vi "Set Results.vi"(8 "error in (no error)":errorcluster, 10 "Results":T1, 11 "niDTS GNSS Dut in":refnum<class "niDTS GNSS Dut.lvclass">) -> (0 "error out":errorcluster, 3 "niDTS GNSS Dut out":refnum<class "niDTS GNSS Dut.lvclass">)   [LabVIEW 2015, in "niDTS GNSS.lvlib" / "niDTS GNSS Dut.lvclass"]
uses:
  niDTS GNSS Dut.lvclass
  Tests/RF Test/Includes/niDTS GNSS RF Test INC Results.ctl
  niDTS GNSS Dut.lvclass/niDTS GNSS Dut.ctl
  niDTS GNSS.lvlib
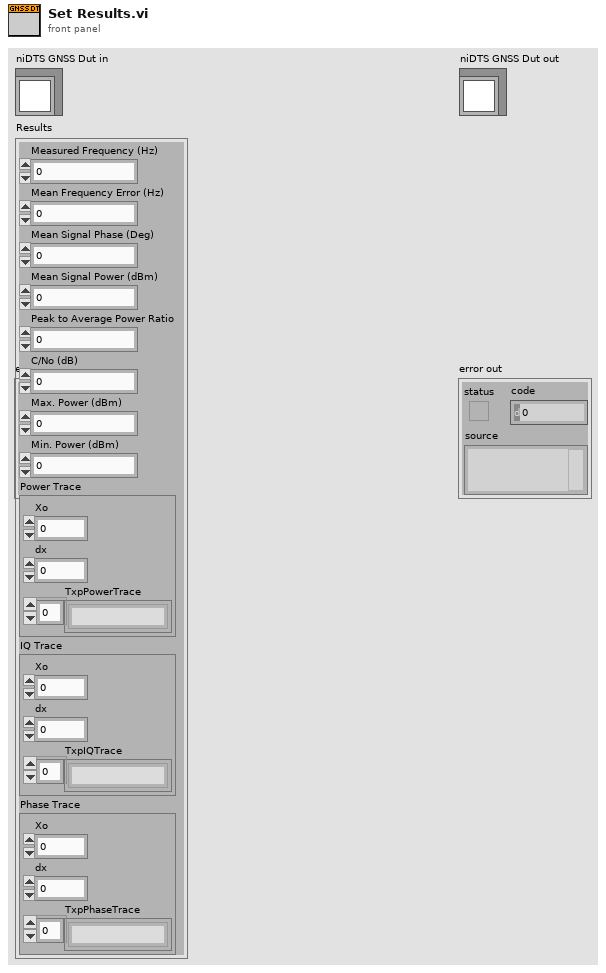
[diagram p1: front panel]
types:
  T1 = typedef "niDTS GNSS.lvlib/niDTS GNSS RF Test INC Results.ctl" = cluster{"Measured Frequency (Hz)":dbl, "Mean Frequency Error (Hz)":dbl, "Mean Signal Phase (Deg)":dbl, "Mean Signal Power (dBm)":dbl, "Peak to Average Power Ratio":dbl, "C/No (dB)":dbl, "Max. Power (dBm)":dbl, "Min. Power (dBm)":dbl, "Power Trace":cluster{"Xo":dbl, "dx":dbl, "TxpPowerTrace":string[]}, "IQ Trace":cluster{"Xo":dbl, "dx":dbl, "TxpIQTrace":string[]}, "Phase Trace":cluster{"Xo":dbl, "dx":dbl, "TxpPhaseTrace":string[]}}
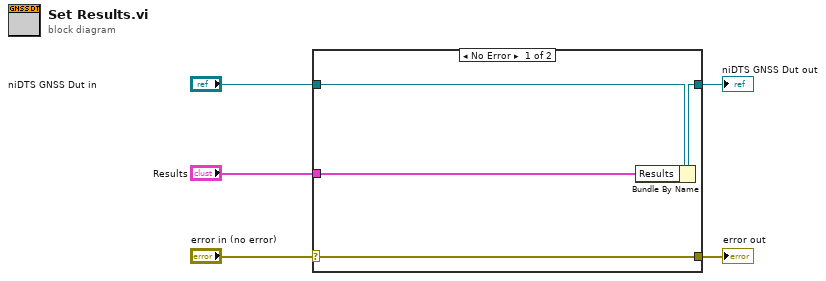
[diagram p0: block diagram]
diagram:
  n1 = case shown="No Error" "error in (no error)" {
    selector: "error in (no error)" -> [w9 w10]
    tunnel: [w9 w10] -> w4
    tunnel: [w7 w11] -> w2
    tunnel: "niDTS GNSS Dut in" -> [w8 w11]
    tunnel: "Results" -> [w6 _]
    frame No Error {
      n2 = Bundle By Name(cluster=w8, "Results"=w6) -> (w7:refnum<class "niDTS GNSS Dut.lvclass">)
    }
    frame Error {
    }
  }
  "error out" <- w4
  "niDTS GNSS Dut out" <- w2
